vi "get-many-videos.vi"() -> ()   [LabVIEW 2024]
uses:
  <vilib>/vision/Avi.llb/IMAQ AVI2 Refnum.ctl
  <vilib>/vision/NI_Vision_Development_Module.lvlib
panel:
  in  "BOOLEAN AI":bool
  out "Path Video":path
  out "Path ADQUISICION":path
  out "USUARIO":string
  out "Boolean":bool
  out "AVI Refnum":T1
  in  "stop 5":bool
  in  "ADQUIRIR":bool
  in  "DETENER":bool
  out "Full Image":T2(plugin-control)
  out "error out":errorcluster
  out "ROI (Ojo)":T2(plugin-control)
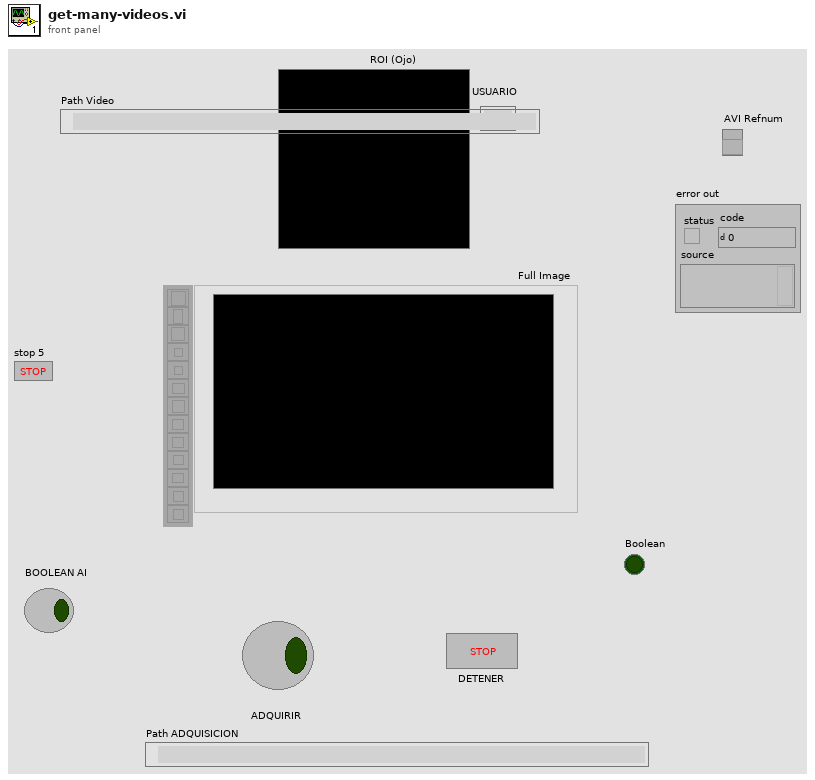
[diagram p1: front panel]
types:
  T1 = typedef "IMAQ AVI2 Refnum.ctl" = refnum<k20>
  T2 = typedef "IMAQ Image.ctl" = refnum<image>
  T3 = typedef "Image Type" = u32
  T4 = cluster{"Global Rectangle":i32[], "Contours":cluster{"Contour Type":u32, "ROI Type":u32, "Points":i32[]}[]}
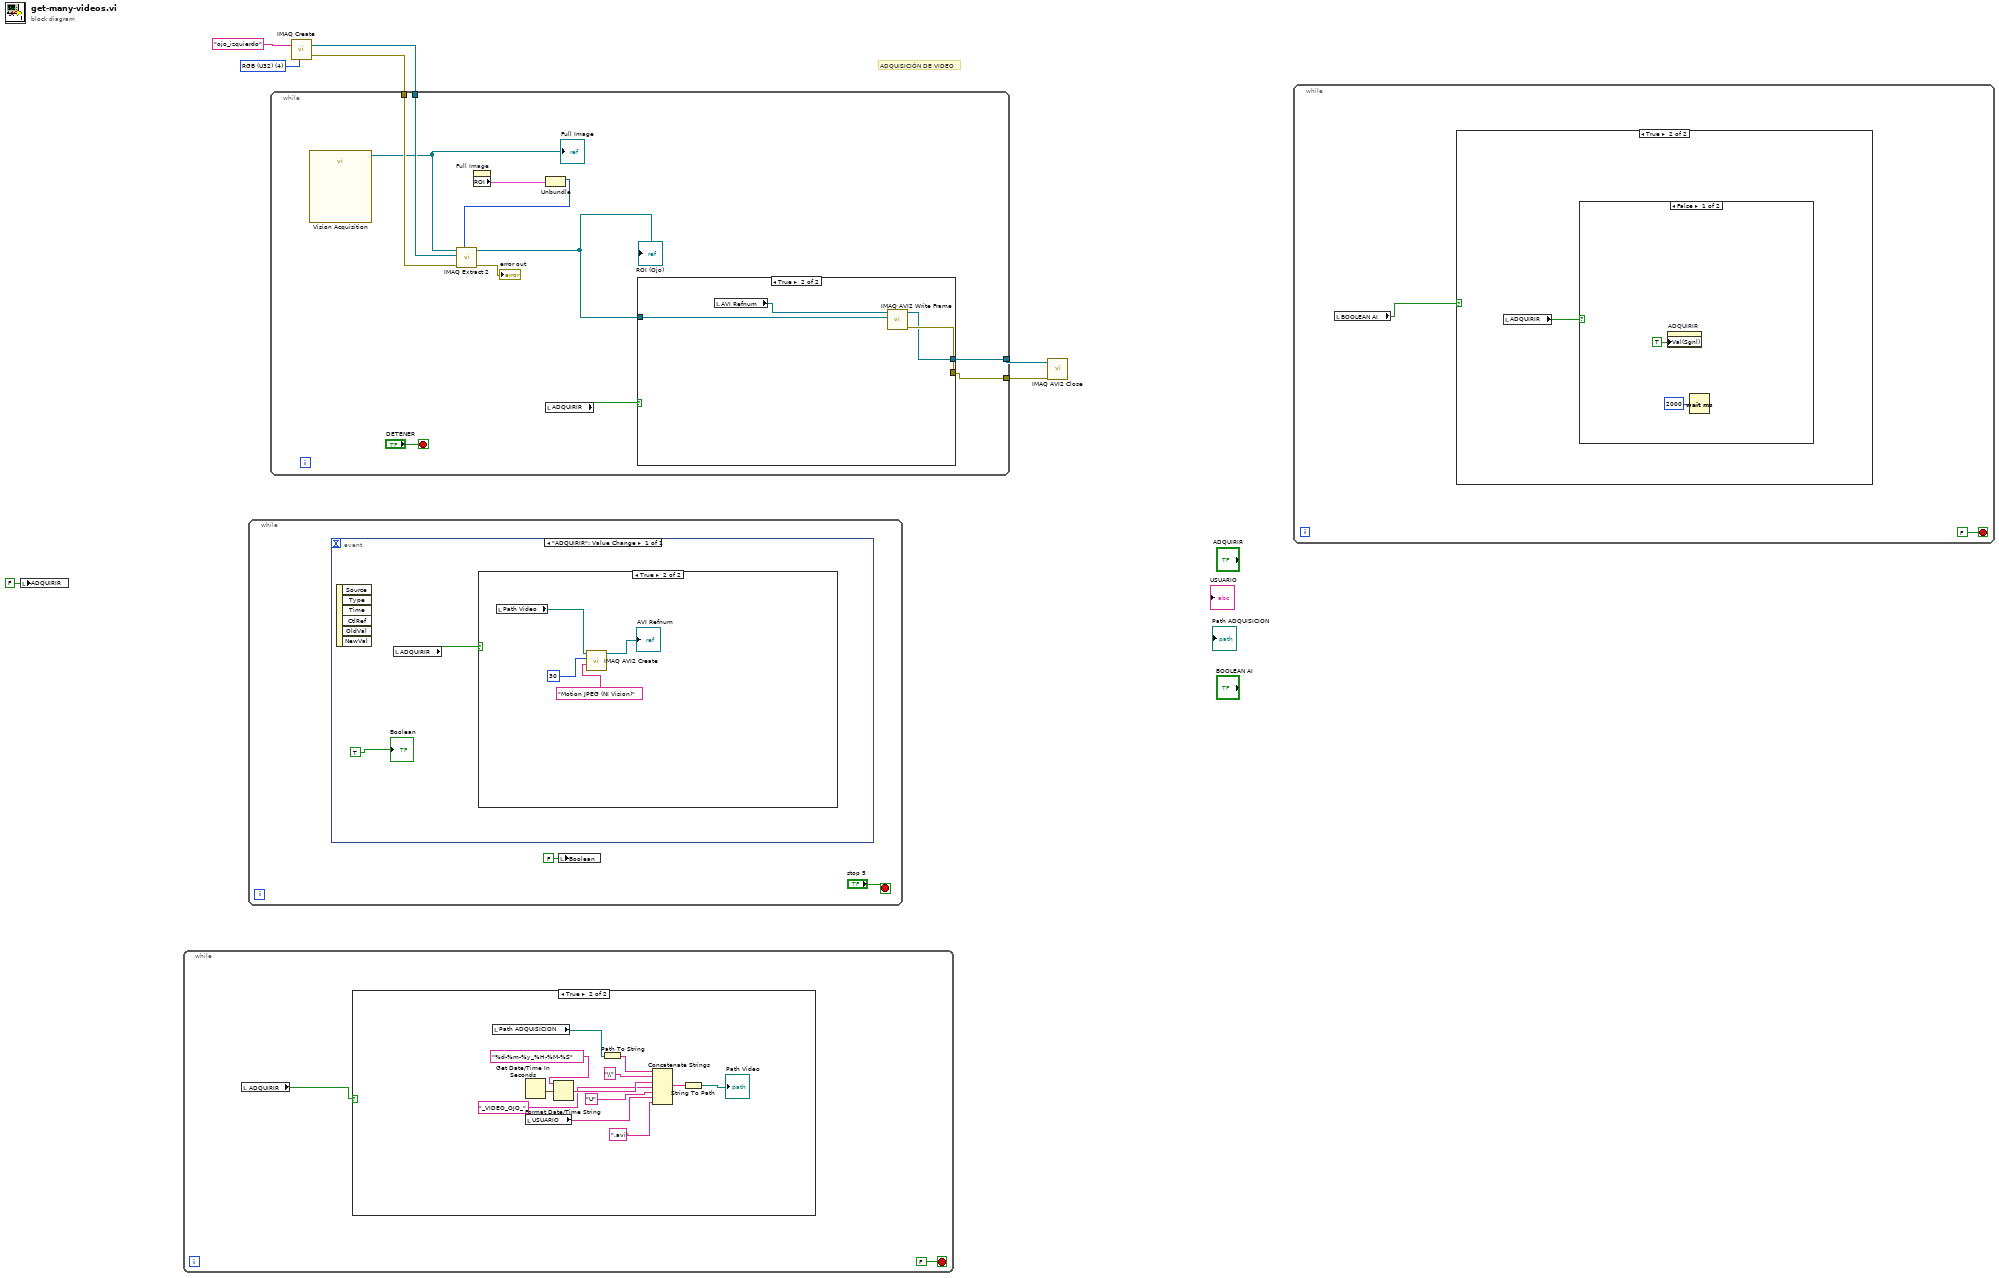
[diagram p0: block diagram]
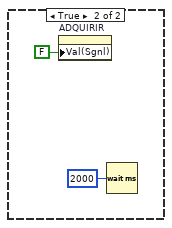
[diagram p3: hidden frame]
diagram:
  w6 = T3 4 items=["Grayscale (U8)", "Grayscale (I16)", "Grayscale (SGL)", "Complex (CSG)", "RGB (U32)", "HSL (U32)", "RGB (U64)", "Grayscale (U16)"] ("Image Type")
  # "ADQUISICIÓN DE VIDEO"
  n1 = local write "ADQUIRIR"(FALSE ("ADQUIRIR")) -> ()
  n2 = while {
    stop <- FALSE stop-if-true
    n3 = local read "ADQUIRIR"() -> (w8:bool)
    n4 = case shown="True" w8 {
      frame False {
      }
      frame True {
        n5 = local read "Path ADQUISICION"() -> (w15:path)
        n6 = Get Date/Time In Seconds() -> (seconds since 1Jan1904=w20:timestamp)
        n7 = local read "USUARIO"() -> (w18:string)
        n8 = Format Date/Time String(time format string (%c)="%d-%m-%y_%H-%M-%S", seconds (now)=w20) -> (date/time string=w19:string)  [unwired: 1 in]
        n9 = Path To String(path=w15) -> (string=w21:string)
        n10 = Concatenate Strings(w21, "\\" ("string"), w19, "_VIDEO_OJO_" ("string"), "U" ("string"), w18, ".avi" ("string")) -> (w17:string)
        n11 = String To Path(string=w17) -> (path=→"Path Video":path)
      }
    }
  }
  n12 = while {
    stop <- "stop 5" stop-if-true
    n13 = event shown="[0] \"ADQUIRIR\": Value Change" {
      selector: _ -> [_]
      dyn-events: _ -> [_]
      timeout: _ -> [_]
      event "ADQUIRIR": Value Change {
        n14 = event-data() -> ()  [unwired: 1 in, 6 out]
        n15 = local read "ADQUIRIR"() -> (w24:bool)
        n16 = case shown="True" w24 {
          frame False {
          }
          frame True {
            n17 = local read "Path Video"() -> (w28:path)
            n18 = call "IMAQ AVI2 Create"("Codec"="Motion JPEG (NI Vision)", "Frames Per Second"=u32 30, "AVI Path"=w28) -> ("AVI Refnum"=→"AVI Refnum":T1)  [unwired: 7 in, 1 out]
          }
        }
        "Boolean" <- TRUE
      }
    }
    n19 = local write "Boolean"(FALSE ("Boolean")) -> ()
  }
  n20 = call "IMAQ Create"("Image Name"="ojo_izquierdo", "Image Type"=w6) -> ("New Image"=w4:T2, "error out"=w5:errorcluster)  [unwired: 3 in]
  n21 = while {
    tunnel: w5 -> [w39]
    tunnel: w4 -> [w38]
    tunnel: [w32] -> w3
    tunnel: [w31] -> w2
    stop <- "DETENER" stop-if-true
    n22 = call "Vision Acquisition"() -> ("Image Out"=w34:T2)  [unwired: 25 in, 2 out]
    "Full Image" <- w34
    n23 = property on="Full Image" class="ImageControl"() -> ("ROI"=w37:T4)  [unwired: 2 in, 2 out]
    n24 = local read "ADQUIRIR"() -> (w30:bool)
    n25 = Unbundle "Unbundle"(w37) -> ("Global Rectangle"=w36:i32[])  [unwired: 1 out]
    n26 = call "IMAQ Extract 2"("Optional Rectangle"=w36, "error in (no error)"=w39, "Image Dst"=w38, "Image Src"=w34) -> ("error out"=→"error out":errorcluster, "Image Dst Out"=w33:T2)  [unwired: 6 in]
    "ROI (Ojo)" <- w33
    n27 = case shown="True" w30 {
      tunnel: [_ w44] -> w32
      tunnel: [_ w43] -> w31
      tunnel: w33 -> [_ w42]
      frame False {
      }
      frame True {
        n28 = local read "AVI Refnum"() -> (w41:T1)
        n29 = call "IMAQ AVI2 Write Frame"("Image"=w42, "AVI Refnum"=w41) -> ("error out"=w44:errorcluster, "AVI Refnum (duplicate)"=w43:T1)  [unwired: 7 in, 1 out]
      }
    }
  }
  n30 = call "IMAQ AVI2 Close"("error in (no error)"=w3, "AVI Refnum"=w2) -> ()  [unwired: 9 in, 1 out]
  n31 = while {
    stop <- FALSE stop-if-true
    n32 = local read "BOOLEAN AI"() -> (w46:bool)
    n33 = case shown="True" w46 {
      frame False {
      }
      frame True {
        n34 = local read "ADQUIRIR"() -> (w47:bool)
        n35 = case shown="False" w47 {
          frame False {
            n36 = property on="ADQUIRIR" class="Bool (strict)"("Val(Sgnl)"=TRUE ("Value (Signaling)")) -> ()  [unwired: 2 in, 2 out]
            n37 = Wait (ms)(milliseconds to wait=u32 2000) -> ()  [unwired: 1 out]
          }
          frame True {
            n38 = property on="ADQUIRIR" class="Bool (strict)"("Val(Sgnl)"=FALSE ("Value (Signaling)")) -> ()  [unwired: 2 in, 2 out]
            n39 = Wait (ms)(milliseconds to wait=u32 2000) -> ()  [unwired: 1 out]
          }
        }
      }
    }
  }
